vi "Write.vi"(8 "error in (no error)":errorcluster, 9 "Device and Axis":string, 10 "Command":string, 11 "VISA resource name":refnum<visa-resource-name>) -> (0 "error out":errorcluster, 3 "VISA resource name out":refnum<visa-resource-name>)   [LabVIEW 2013, in "Zaber A Series.lvlib"]
doc: "Writes a string to the serial port. The communication protocol is detailed at http://www.zaber.com/wiki/Manuals/ASCII_Protocol_Manual. The complete command should be sent to the Command input, but you can optionally input the Device and Axis separately and the VI will bundle these. Additionally the VI will add the required prefix and terminator for the command. \n\nThis VI requires that the Initialize VI has been called with the same serial port."
uses:
  Zaber A Series.lvlib
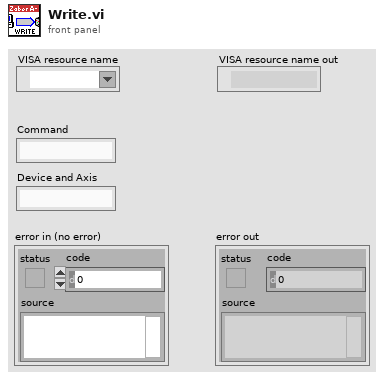
[diagram p1: front panel]
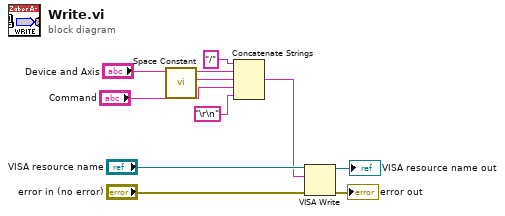
[diagram p0: block diagram]
diagram:
  n1 = call <vilib>:"Space Constant.vi"() -> ("String"=w3:string)
  n2 = Concatenate Strings("/" ("string"), "Device and Axis", w3, "Command", "\r\n") -> (w4:string)
  n3 = VISA Write(VISA resource name="VISA resource name", write buffer=w4, error in (no error)="error in (no error)") -> (VISA resource name out=→"VISA resource name out":refnum<visa-resource-name>, error out=→"error out":errorcluster)  [unwired: 1 out]
